vi "Init.vi"(8 "error in (no error)":errorcluster, 10 "Instrument String":variant, 11 "NI DIO in":refnum<class "NI DIO.lvclass">) -> (0 "error out":errorcluster, 2 "Found?":bool=TRUE, 3 "NI DIO out":refnum<class "NI DIO.lvclass">)   [LabVIEW 2025, in "Digital IO.lvlib" / "NI DIO.lvclass"]
uses:
  NI DIO.lvclass
  C:/Working copy/tss/Plugin/Engines/Digital IO/Digital IO Instrument/Digital IO Instrument.lvclass
  Users/Public/Documents/Sandia National Labs/TSS Plugin/Abstract Engine.lvlibp/Plugin/Abstract/Instrument configuration/Instrument configuration.lvclass
  NI DIO.lvclass/NI DIO.ctl
  Users/Public/Documents/Sandia National Labs/TSS Plugin/Abstract Engine.lvlibp/Plugin/Abstract/Instrument configuration/Read Instrument Setting.vi
  <vilib>/DAQmx/create/channels.llb/DAQmx Create Channel (DO-Digital Output).vi
  Users/Public/Documents/Sandia National Labs/TSS Plugin/CEF.lvlibp/serializable configuration/CEF_serializable configuration.lvclass
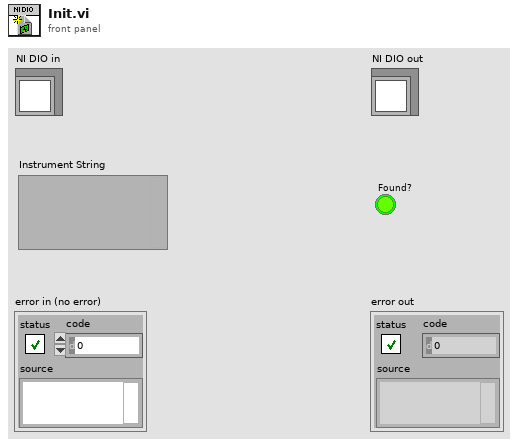
[diagram p1: front panel]
types:
  T1 = cluster{"Type":string, "Engine IP Address":string, "Engine Port":u32, "Address":string, "SW Alias":string, "Description":string, "Enabled":bool, "Model":string, "Serial Number":string, "Asset Number":string, "Calibration Date":string}
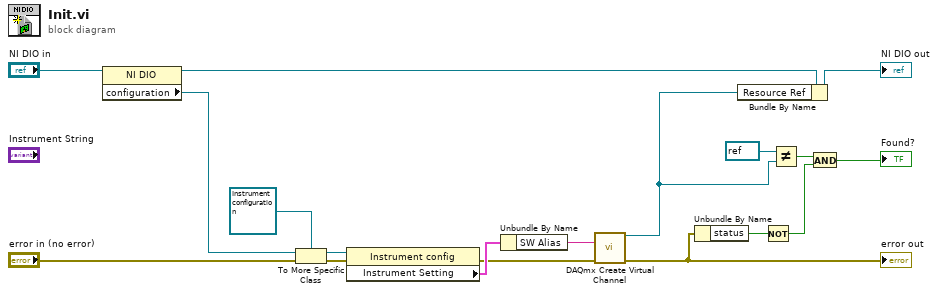
[diagram p0: block diagram]
diagram:
  n1 = property class="NI DIO"(reference="NI DIO in") -> (reference out=w16:refnum<class "NI DIO.lvclass">, "configuration"=w14:refnum<class "CEF_serializable configuration.lvclass">)  [unwired: 1 in, 1 out]
  n2 = To More Specific Class(target class=refnum<class "Instrument configuration.lvclass"> refnum ("Abstract PlugIn.lvlibp:Instrument config"), reference=w14, error in="error in (no error)") -> (specific class reference=w15:refnum<class "Instrument configuration.lvclass">, error out=w12:errorcluster)
  n3 = property class="Instrument config"(reference=w15, error in=w12) -> (error out=w8:errorcluster, "Instrument Setting"=w11:T1)  [unwired: 1 out]
  n4 = Unbundle By Name(w11) -> ("SW Alias"=w6:string)
  n5 = call-poly <vilib>:"DAQmx Create Virtual Channel.vi"("lines"=w6, "error in"=w8) -> ("task out"=w5:refnum<k21>, "error out"=w7:errorcluster)  [unwired: 12 in]
  "error out" <- w7
  n6 = Unbundle By Name(w7) -> ("status"=w10:bool)
  n7 = Bundle By Name(cluster=w16, "Resource Ref"=w5) -> (→"NI DIO out":refnum<class "NI DIO.lvclass">)
  n8 = Not(x=w10) -> (.not. x?=w9:bool)
  n9 = Not Equal?(x=refnum<k21> refnum, y=w5) -> (x != y?=w3:bool)
  n10 = And(x=w3, y=w9) -> (x .and. y?=→"Found?":bool)
